vi "read.vi"(8 "error in (no error)":errorcluster, 11 "SerialSimulator in":refnum<class "SerialSimulator.lvclass">) -> (0 "error out":errorcluster, 2 "stringRead":string, 3 "SerialSimulator out":refnum<class "SerialSimulator.lvclass">)   [LabVIEW 2013, in "SerialProtocols.lvlib" / "SerialSimulator.lvclass"]
uses:
  <userlib>/Common/SerialProtocols/SerialCommunicator/SerialSimulator/SerialSimulator.lvclass
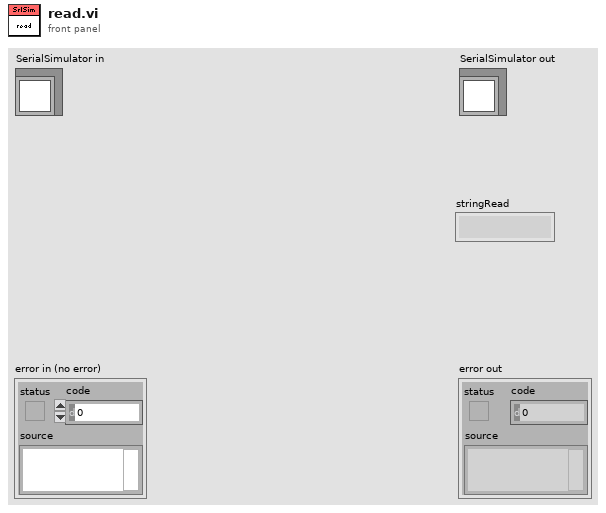
[diagram p1: front panel]
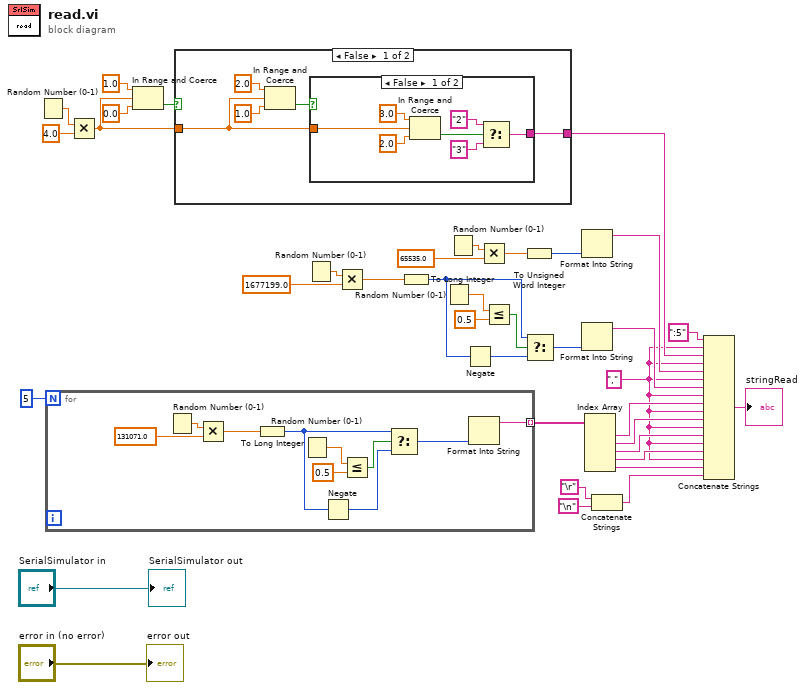
[diagram p0: block diagram]
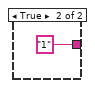
[diagram p2: hidden frame]
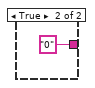
[diagram p3: hidden frame]
diagram:
  w3 = "," ("string")
  n1 = Random Number (0-1)() -> (number: 0 to 1=w34:dbl)
  n2 = for {
    N: 5 -> [_]
    tunnel: [w38] -> w8 mode=indexing
    n3 = Random Number (0-1)() -> (number: 0 to 1=w39:dbl)
    n4 = Multiply(x=w39, y=131071.0) -> (x*y=w43:dbl)
    n5 = To Long Integer(number=w43) -> (32bit integer=w44:i32)
    n6 = Random Number (0-1)() -> (number: 0 to 1=w41:dbl)
    n7 = Negate(x=w44) -> (-x=w46:i32)
    n8 = Less Or Equal?(x=w41, y=0.5) -> (x <= y?=w45:bool)
    n9 = Select(t=w44, s=w45, f=w46) -> (s? t:f=w47:i32)
    n10 = Format Into String(w47) -> (resulting string=w38:string)  [unwired: 3 in, 1 out]
  }
  n11 = Multiply(x=w34, y=4.0) -> (x*y=w1:dbl)
  n12 = In Range and Coerce(upper limit=1.0, x=w1, lower limit=0.0) -> (In Range?=w30:bool)  [unwired: 1 out]
  n13 = case shown="False" w30 {
    tunnel: [w49 "0" ("string")] -> w29
    tunnel: w1 -> [w48 _]
    frame False {
      n14 = In Range and Coerce(upper limit=2.0, x=w48, lower limit=1.0) -> (In Range?=w50:bool)  [unwired: 1 out]
      n15 = case shown="False" w50 {
        tunnel: [w54 "1" ("string")] -> w49
        tunnel: w48 -> [w53 _]
        frame False {
          n16 = In Range and Coerce(upper limit=3.0, x=w53, lower limit=2.0) -> (In Range?=w57:bool)  [unwired: 1 out]
          n17 = Select(t="2" ("string"), s=w57, f="3" ("string")) -> (s? t:f=w54:string)
        }
        frame True {
        }
      }
    }
    frame True {
    }
  }
  n18 = Random Number (0-1)() -> (number: 0 to 1=w22:dbl)
  n19 = Multiply(x=w22, y=1677199.0) -> (x*y=w18:dbl)
  n20 = To Long Integer(number=w18) -> (32bit integer=w17:i32)
  n21 = Random Number (0-1)() -> (number: 0 to 1=w20:dbl)
  n22 = Random Number (0-1)() -> (number: 0 to 1=w26:dbl)
  n23 = Negate(x=w17) -> (-x=w15:i32)
  n24 = Multiply(x=w26, y=65535.0) -> (x*y=w25:dbl)
  n25 = Less Or Equal?(x=w20, y=0.5) -> (x <= y?=w16:bool)
  n26 = To Unsigned Word Integer(number=w25) -> (unsigned 16bit integer=w24:u16)
  n27 = Select(t=w17, s=w16, f=w15) -> (s? t:f=w14:i32)
  n28 = Format Into String(w24) -> (resulting string=w23:string)  [unwired: 3 in, 1 out]
  n29 = Format Into String(w14) -> (resulting string=w13:string)  [unwired: 3 in, 1 out]
  n30 = Index Array(array=w8) -> (element #1=w7:string, element #2=w6:string, element #3=w5:string, element #4=w4:string, element #5=w2:string)  [unwired: 5 in]
  n31 = Concatenate Strings("\r", "\n") -> (w10:string)
  n32 = Concatenate Strings(":5" ("string"), w3, w29, w3, w23, w3, w13, w3, w7, w3, w6, w3, w5, w3, w4, w3, w2, w10) -> (→"stringRead":string)
  "error out" <- "error in (no error)"
  "SerialSimulator out" <- "SerialSimulator in"
